vi "TempLogger_SaveData.vi"(10 "Data":dbl[](array[numeric]), 11 "element":T1) -> (0 "error out":errorcluster)   [LabVIEW 2022 SP3]
uses:
  <vilib>/Utility/file.llb/Write Delimited Spreadsheet (DBL).vi
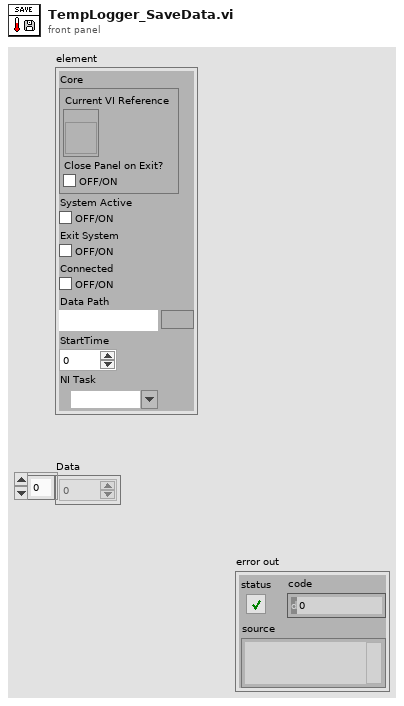
[diagram p1: front panel]
types:
  T1 = cluster{"Core":cluster{"Current VI Reference":refnum<vi>, "Close Panel on Exit?":bool}, "System Active":bool, "Exit System":bool, "Connected":bool, "Data Path":path, "StartTime":u32, "NI Task":refnum<k21>}
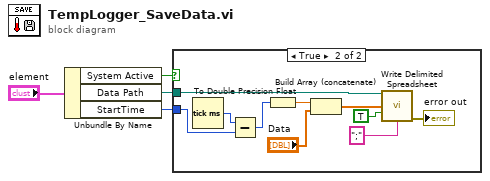
[diagram p0: block diagram]
diagram:
  n1 = Unbundle By Name("element") -> ("System Active"=w1:bool, "Data Path"=w2:path, "StartTime"=w3:u32)
  n2 = case shown="True" w1 {
    tunnel: w3 -> [_ w9]
    tunnel: w2 -> [_ w6]
    frame False {
    }
    frame True {
      n3 = Tick Count (ms)() -> (millisecond timer value=w14:u32)
      n4 = Subtract(x=w14, y=w9) -> (x-y=w10:u32)
      n5 = To Double Precision Float(number=w10) -> (double precision float=w13:dbl)
      n6 = Build Array (concatenate)(w13, "Data") -> (w12:dbl[])
      n7 = call-poly <vilib>:"Write Delimited Spreadsheet.vi"("file path (dialog if empty)"=w6, "1D data"=w12, "append to file? (new file:F)"=TRUE, "delimiter (\\t)"=";" ("delimiter (\\t)")) -> ("error out"=→"error out":errorcluster)  [unwired: 10 in, 1 out]
    }
  }
